vi "LKIF2_DataStorageGetData.vi"(8 "error in (no error)":errorcluster {"code" format="%x"}, 10 "NumOutBuffer":i32=1, 11 "OutNo (0: OUT1)":i32) -> (0 "error out":errorcluster {"code" format="%x"}, 2 "NumReceived":i32, 3 "OutBuffer":T1[](array[typedef]) {"LKIF_FLOATRESULT" items=["VALID", "RANGEOVER_P", "RANGEOVER_N", "WAITING", "ALARM", "INVALID"]})   [LabVIEW 2013, in "Keyence LK-G5000.lvlib"]
uses:
  <instrlib>/Keyence LK-G5000/Keyence LK-G5000.lvlib
  <instrlib>/Keyence LK-G5000/Public/Clusters/LKIF_FLOATVALUE.ctl
  <instrlib>/Keyence LK-G5000/Public/enum/LKIF_FLOATRESULT.ctl
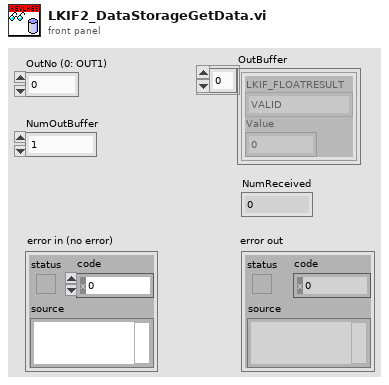
[diagram p1: front panel]
types:
  T1 = typedef "Keyence LK-G5000.lvlib/LKIF_FLOATVALUE.ctl" = cluster{"LKIF_FLOATRESULT":T2, "Value":sgl}
  T2 = typedef "Keyence LK-G5000.lvlib/LKIF_FLOATRESULT.ctl" = i32
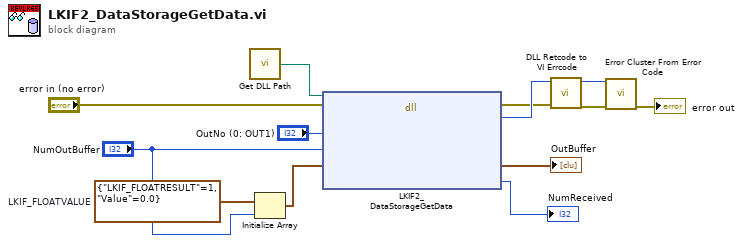
[diagram p0: block diagram]
diagram:
  w9 = T1 {"LKIF_FLOATRESULT"=1, "Value"=0.0}  # LKIF_FLOATVALUE
  n1 = call <instrlib>:"Get DLL Path.vi"() -> ("DLL Path"=w1:path)  [unwired: 1 in]
  n2 = Initialize Array(w9, "NumOutBuffer") -> (w8:T1[])
  n3 = dll-call lib="C:/Program Files/National Instruments/LabVIEW 2011/instr.lib/Keyence LK-G5000/LKIF2.dll" fn="LKIF2_DataStorageGetData"(path in=w1, error in="error in (no error)", "OutNo"="OutNo (0: OUT1)", "NumOutBuffer"="NumOutBuffer", "OutBuffer"=w8) -> (error out=w3:errorcluster, "RC"=w4:i32, "OutBuffer"=→"OutBuffer":T1[], "NumReceived"=→"NumReceived":i32)  [unwired: 4 in, 1 out]
  n4 = call <instrlib>:"DLL Retcode to VI Errcode.vi"("error in (no error)"=w3, "DLL Retcode"=w4) -> ("error out"=w13:errorcluster, "VI Errcode"=w12:i32)  [unwired: 8 in]
  n5 = call <vilib>:"Error Cluster From Error Code.vi"("error in (no error)"=w13, "error code (0)"=w12) -> ("error out"=→"error out":errorcluster)  [unwired: 7 in]
